vi "AODO-Wait To Write.vi"(0 "Tnext in":dbl format="%#_16g", 2 "Headway":dbl, 5 "Parse End Queue In":refnum<queue>, 9 "Poll (s)":dbl, 11 "error in (no error)":errorcluster, 12 "Frame size":i32) -> (4 "Tnext out":dbl format="%#_16g", 15 "error out":errorcluster)   [LabVIEW 2015]
uses:
  Tosca/LV Source/Typedefs/Tosca-End Parser Queue Data.ctl
  Typedefs/AODO-Action.ctl
  TDT VIs/TDT AODO VIs/Typedefs/TDT-AODO-Action.ctl
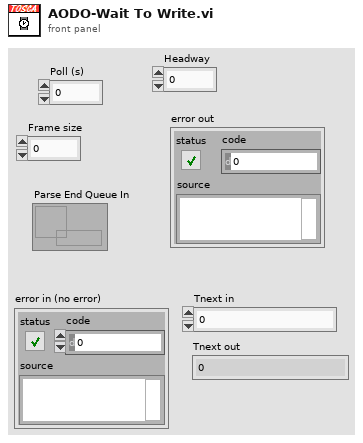
[diagram p1: front panel]
types:
  T1 = typedef "AODO-Action.ctl" = enum16{"Configure", "Initialize", "Start", "Write", "Clean up", "Init & Start", "Config & Test", "Position", "Set AO Gains"}
  T2 = typedef "TDT-AODO-Action.ctl" = enum16{"Configure", "Initialize", "Start", "Stop", "Write", "Clean up", "Space available"}
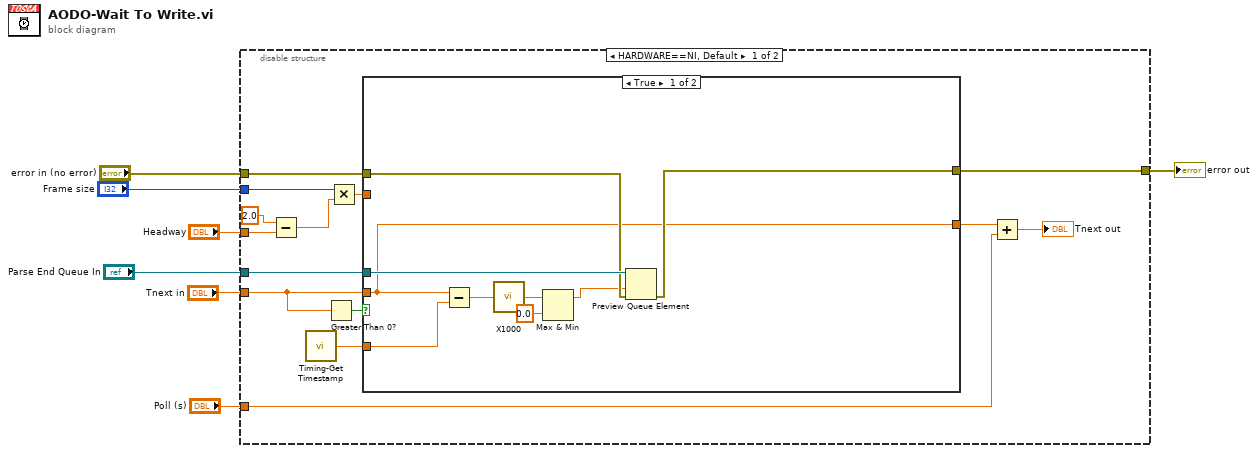
[diagram p0: block diagram]
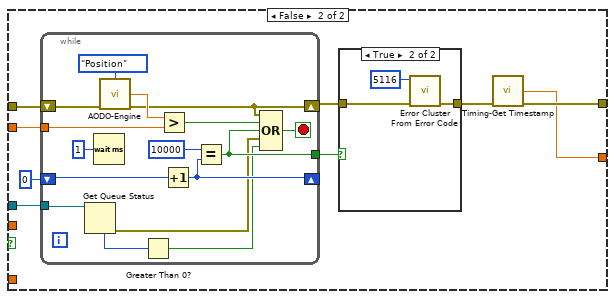
[diagram p2: hidden frame]
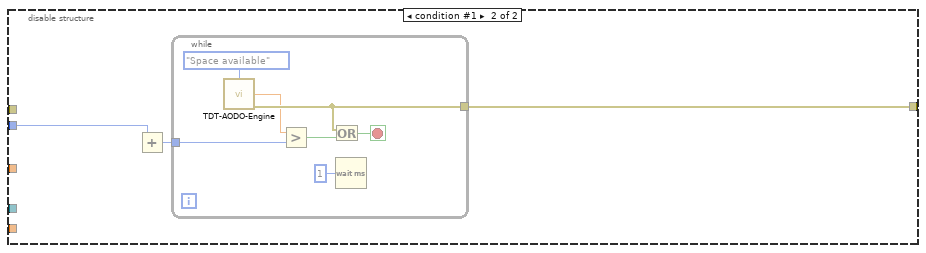
[diagram p4: hidden frame]
diagram:
  n1 = disable-structure shown="HARDWARE==NI, Default" {
    disable-tunnel: [w21 w62] -> w4
    disable-tunnel: "Frame size" -> [w12 w61]
    disable-tunnel: "Parse End Queue In" -> [w20 _]
    disable-tunnel: "error in (no error)" -> [w19 _]
    disable-tunnel: "Tnext in" -> [w15 _]
    disable-tunnel: "Poll (s)" -> [w13 _]
    disable-tunnel: "Headway" -> [w10 _]
    frame condition #0 (active) {
      n2 = Subtract(x=2.0, y=w10) -> (x-y=w9:dbl)
      n3 = call "Timing-Get Timestamp.vi"() -> ("double precision float"=w17:dbl)  [unwired: 14 in, 1 out]
      n4 = Greater Than 0?(x=w15) -> (x > 0?=w16:bool)
      n5 = Multiply(x=w12, y=w9) -> (x*y=w11:dbl)
      n6 = case shown="True" w16 {
        tunnel: w11 -> [_ w39]
        tunnel: [w27 w33] -> w21
        tunnel: w20 -> [w30 w36]
        tunnel: w19 -> [w29 w35]
        tunnel: [w24 w32] -> w18
        tunnel: w17 -> [w26 _]
        tunnel: w15 -> [w24 _]
        frame True {
          n7 = Subtract(x=w24, y=w26) -> (x-y=w28:dbl)
          n8 = call "X1000.vi"("X"=w28) -> ("X/1000"=w25:dbl)
          n9 = Max & Min(x=w25, y=0.0) -> (max(x,y)=w23:dbl)  [unwired: 1 out]
          n10 = Preview Queue Element(queue=w30, timeout in ms (-1)=w23, error in (no error)=w29) -> (error out=w27:errorcluster)  [unwired: 3 out]
        }
        frame False {
          n11 = while {
            tunnel: w39 -> [w57]
            shift-right: [w52] -> _
            shift-left: 0 -> [w53]
            tunnel: [w50] -> w38
            tunnel: w36 -> [w49]
            shift-right: [w56] -> w37
            shift-left: w35 -> [w45]
            stop <- w54 stop-if-true
            n12 = Get Queue Status(queue=w49) -> (error out=w46:errorcluster, # elements in queue=w48:i32)  [unwired: 2 in, 6 out]
            n13 = Wait (ms)(milliseconds to wait=u32 1) -> ()  [unwired: 1 out]
            n14 = call "AODO-Engine.vi"("Action"=AODO-Action."Position", "error in (no error)"=w45) -> ("Position"=w58:dbl, "error out"=w56:errorcluster)  [unwired: 12 in]
            n15 = Greater Than 0?(x=w48) -> (x > 0?=w47:bool)
            n16 = Greater?(x=w58, y=w57) -> (0:w55:bool)
            n17 = Increment(x=w53) -> (x+1=w52:i32)
            n18 = Equal?(x=10000, y=w52) -> (x = y?=w50:bool)
            n19 = Compound Arithmetic op=OR(w56, w55, w50, w46, w47) -> (w54:bool)
          }
          n20 = case shown="True" w38 {
            tunnel: w37 -> [w40 w43]
            tunnel: [w40 w42] -> w34
            frame False {
            }
            frame True {
              n21 = call <vilib>:"Error Cluster From Error Code.vi"("error in (no error)"=w43, "error code (0)"=5116) -> ("error out"=w42:errorcluster)  [unwired: 7 in]
            }
          }
          n22 = call "Timing-Get Timestamp.vi"("error in (no error)"=w34) -> ("double precision float"=w32:dbl, "error out"=w33:errorcluster)  [unwired: 13 in]
        }
      }
      n23 = Add(x=w18, y=w13) -> (x+y=→"Tnext out":dbl)
    }
    frame condition #1 {
      n24 = Add(x=w61) -> (x+y=w60:i32)  [unwired: 1 in]
      n25 = while {
        tunnel: [w66] -> w62
        tunnel: w60 -> [w64]
        stop <- w67 stop-if-true
        n26 = call "TDT-AODO-Engine.vi"("Action"=TDT-AODO-Action."Space available") -> ("Space Available"=w63:dbl, "error out"=w66:errorcluster)  [unwired: 12 in, 1 out]
        n27 = Greater?(x=w63, y=w64) -> (0:w68:bool)
        n28 = Or(x=w66, y=w68) -> (x .or. y?=w67:bool)
        n29 = Wait (ms)(milliseconds to wait=u32 1) -> ()  [unwired: 1 out]
      }
    }
  }
  "error out" <- w4
